vi "-8480 Channel unavailable--error.vi"(8 "error in (no error)":errorcluster, 11 "Channel":string) -> (0 "error out":errorcluster)   [LabVIEW 2024, in "PCAN.lvlib" / "PCAN.lvclass"]
uses:
  PCAN.lvclass
  PCAN.lvclass/PCAN.ctl
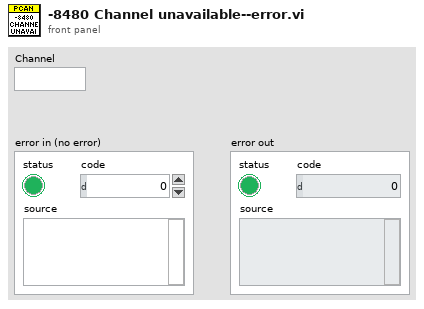
[diagram p1: front panel]
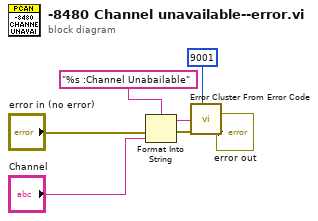
[diagram p0: block diagram]
diagram:
  n1 = Format Into String(format string="%s :Channel Unabailable" ("source"), error in="error in (no error)", "Channel") -> (resulting string=w6:string, error out=w5:errorcluster)  [unwired: 1 in]
  n2 = call <vilib>:"Error Cluster From Error Code.vi"("error in (no error)"=w5, "error message (\"\")"=w6, "error code (0)"=9001) -> ("error out"=→"error out":errorcluster)  [unwired: 6 in]
